vi "CreatePinmapWith3Pins_QueryPins_3PinsFound.vi"() -> (6 "pass":bool, 8 "result":string, 15 "error out":errorcluster)   [LabVIEW 2020]
uses:
  Pin Map Client_v1/RPC Messages/ni_measurementlink_pinmap_v1_CreatePinMapFromXmlRequest.ctl
  Pin Map Client_v1/RPC Messages/ni_measurementlink_pinmap_v1_QueryPinsRequest.ctl
  Pin Map Client_v1/Pin Map Client_v1.lvlib
panel:
  # "Test assumes discovery service and pin map service has already been started."
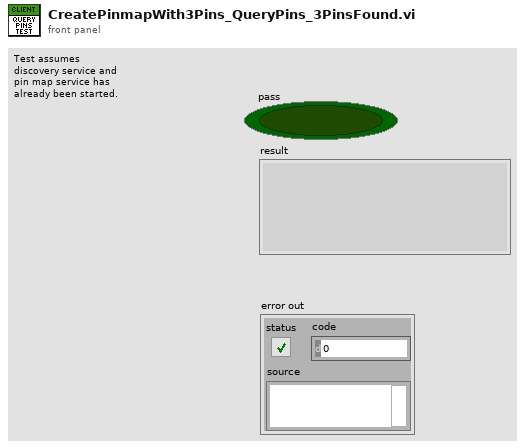
[diagram p1: front panel]
types:
  T1 = typedef "Pin Map Client_v1.lvlib/ni_measurementlink_pinmap_v1_QueryPinsRequest.ctl" = cluster{"pin_map_id":string, "instrument_type_id":string}
  T2 = typedef "Pin Map Client_v1.lvlib/ni_measurementlink_pinmap_v1_CreatePinMapFromXmlRequest.ctl" = cluster{"pin_map_id":string, "pin_map_xml":string}
  T3 = typedef "grpc-lvsupport-release.lvlib/grpcId.ctl" = u64
  T4 = typedef "Pin Map Client_v1.lvlib/ni_measurementlink_pinmap_v1_PinMap.ctl" = cluster{"pin_map_id":string}
  T5 = typedef "Pin Map Client_v1.lvlib/ni_measurementlink_pinmap_v1_QueryPinsResponse.ctl" = cluster{"pins":T6[], "pin_groups":T7[]}
  T6 = typedef "Pin Map Client_v1.lvlib/ni_measurementlink_pinmap_v1_QueryPinsResponse_PinDefinition.ctl" = cluster{"display_name":string, "is_system_pin":bool}
  T7 = typedef "Pin Map Client_v1.lvlib/ni_measurementlink_pinmap_v1_QueryPinsResponse_PinGroupDefinition.ctl" = cluster{"display_name":string, "pin_or_group_references":string[], "resolved_pins":string[]}
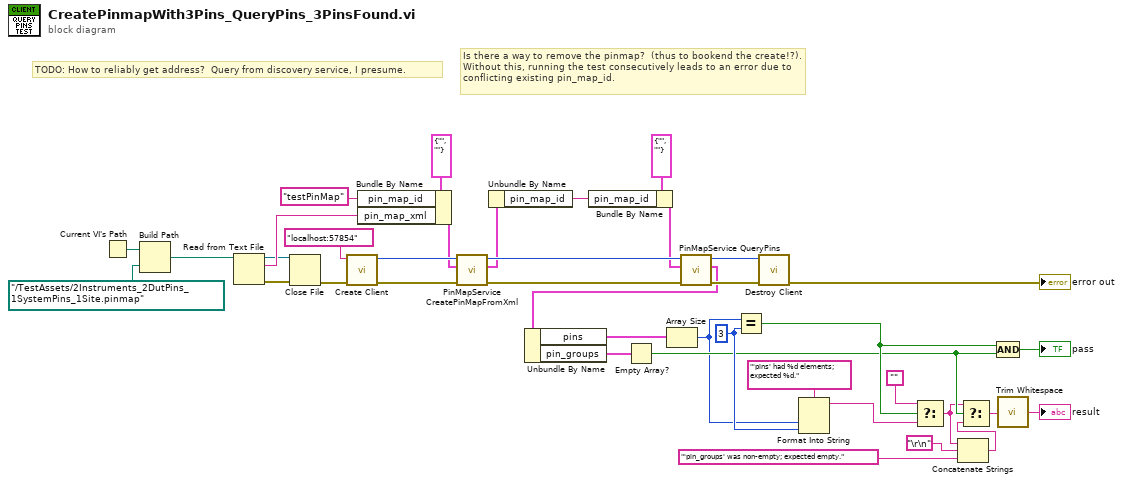
[diagram p0: block diagram]
diagram:
  w13 = 3 ("y")
  # "TODO: How to reliably get address?  Query from discovery service, I presume."
  # "Is there a way to remove the pinmap?  (thus to bookend the create!?).  Without this, running the test consecutively leads to an error due to conflicting existing pin_map_id."
  n1 = Current VI's Path() -> (path=w35:path)
  n2 = Build Path(base path=w35, name or relative path=path "../TestAssets/2Instruments_2DutPins_1SystemPins_1Site.pinmap") -> (appended path=w33:path)
  n3 = Read from Text File(file (use dialog)=w33) -> (refnum out=w29:refnum<file>, text=w31:string, error out=w30:errorcluster)  [unwired: 3 in, 1 out]
  n4 = Close File(refnum=w29, error in=w30) -> (error out=w28:errorcluster)  [unwired: 1 out]
  n5 = call "Create Client.vi"("error in"=w28, "address"="localhost:57854") -> ("error out"=w37:errorcluster, "gRPC ID Out"=w36:T3)  [unwired: 8 in]
  n6 = Bundle By Name(cluster=T2 {"pin_map_id"="", "pin_map_xml"=""} ("Request Data"), "pin_map_id"="testPinMap", "pin_map_xml"=w31) -> (w27:T2)
  n7 = call "PinMapService CreatePinMapFromXml.vi"("error in"=w37, "Request Data"=w27, "gRPC ID"=w36) -> ("error out"=w25:errorcluster, "Response Data"=w19:T4, "gRPC ID out"=w26:T3)  [unwired: 6 in]
  n8 = Unbundle By Name(w19) -> ("pin_map_id"=w20:string)
  n9 = Bundle By Name(cluster=T1 {"pin_map_id"="", "instrument_type_id"=""} ("Request Data"), "pin_map_id"=w20) -> (w18:T1)
  n10 = call "PinMapService QueryPins.vi"("error in"=w25, "Request Data"=w18, "gRPC ID"=w26) -> ("error out"=w24:errorcluster, "Response Data"=w17:T5, "gRPC ID out"=w23:T3)  [unwired: 6 in]
  n11 = Unbundle By Name(w17) -> ("pins"=w16:T6[], "pin_groups"=w2:T7[])
  n12 = Empty Array?(array=w2) -> (empty?=w9:bool)
  n13 = Array Size(array=w16) -> (size(s)=w1:i32)
  n14 = Equal?(x=w1, y=w13) -> (x = y?=w12:bool)
  n15 = call "Destroy Client.vi"("error in"=w24, "gRPC ID"=w23) -> ("error out"=→"error out":errorcluster)  [unwired: 9 in]
  n16 = Format Into String(format string="'pins' had %d elements; expected %d.", w1, w13) -> (resulting string=w11:string)  [unwired: 2 in, 1 out]
  n17 = Select(t="", s=w12, f=w11) -> (s? t:f=w5:string)
  n18 = Concatenate Strings(w5, "\r\n", "'pin_groups' was non-empty; expected empty.") -> (w8:string)
  n19 = Select(t=w5, s=w9, f=w8) -> (s? t:f=w4:string)
  n20 = Compound Arithmetic op=AND(w12, w9) -> (→"pass":bool)
  n21 = call <vilib>:"Trim Whitespace.vi"("string"=w4) -> ("trimmed string"=→"result":string)  [unwired: 1 in]
